vi "draw.vi"(8 "error in (no error)":errorcluster, 11 "Dot in":refnum<class "Dot.lvclass">) -> (0 "error out":errorcluster, 3 "Dot out":refnum<class "Dot.lvclass">)   [LabVIEW 2017, in "Dot.lvclass"]
uses:
  Dot.lvclass
  Shape Class/Shape.lvclass
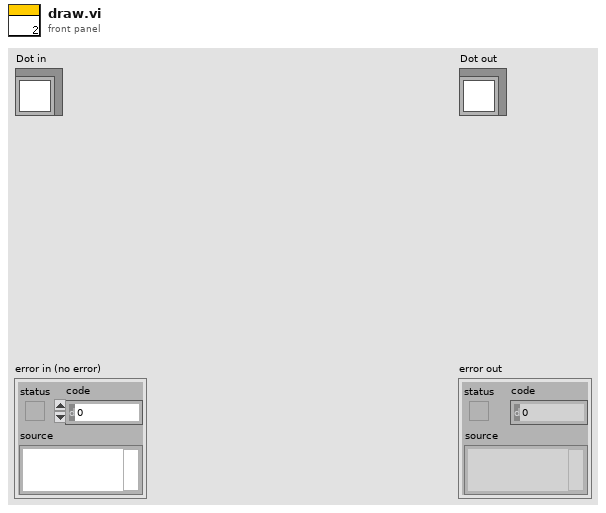
[diagram p1: front panel]
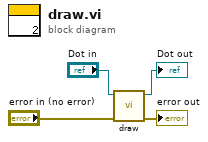
[diagram p0: block diagram]
diagram:
  n1 = call-parent "draw.vi"("error in (no error)"="error in (no error)", "Shape in"="Dot in") -> ("error out"=→"error out":errorcluster, "Shape out"=→"Dot out":refnum<class "Dot.lvclass">)  [unwired: 8 in]
